vi "8.9.1.vi"() -> ()   [LabVIEW 2018]
panel:
  in  "정지":bool
  in  "데이터송신":bool
  out "수신 데이터":string
  in  "송신 데이터":string
  out "슬레이브 루프 반복":dbl
  out "마스터 루프 반복":dbl
  # "송신"
  # "송신안함"
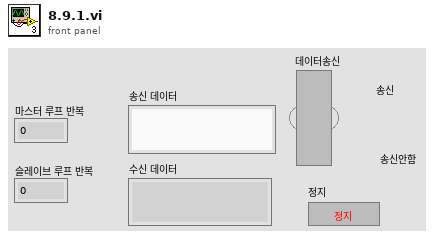
[diagram p1: front panel]
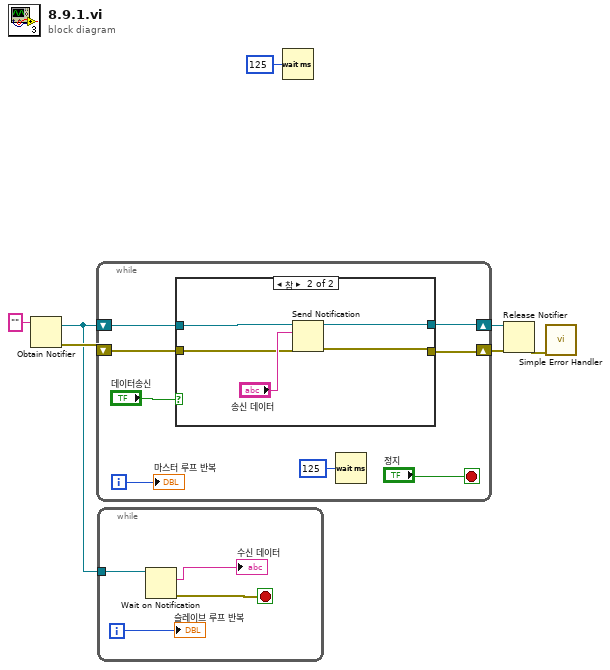
[diagram p0: block diagram]
diagram:
  n1 = Obtain Notifier(notification data type="" ("송신 데이터")) -> (notifier out=w1:refnum<notifier>, error out=w3:errorcluster)  [unwired: 3 in, 1 out]
  n2 = while {
    shift-right: [w11] -> w4
    shift-left: w1 -> [w12]
    shift-right: [w9] -> w2
    shift-left: w3 -> [w10]
    i -> [w15]
    stop <- "정지" stop-if-true
    n3 = case shown="참" "데이터송신" {
      tunnel: w12 -> [w17 w21]
      tunnel: [w17 w20] -> w11
      tunnel: w10 -> [w16 w19]
      tunnel: [w16 w18] -> w9
      frame False {
      }
      frame True {
        n4 = Send Notification(notification="송신 데이터", notifier=w21, error in (no error)=w19) -> (notifier out=w20:refnum<notifier>, error out=w18:errorcluster)
      }
    }
    n5 = Wait (ms)(milliseconds to wait=u32 125 ("대기 시간 (ms)")) -> ()  [unwired: 1 out]
    "마스터 루프 반복" <- w15
  }
  n6 = while {
    tunnel: w1 -> [w23]
    i -> [w26]
    stop <- w25 stop-if-true
    n7 = Wait on Notification(notifier=w23) -> (notification=→"수신 데이터":string, error out=w25:errorcluster)  [unwired: 3 in, 2 out]
    "슬레이브 루프 반복" <- w26
  }
  n8 = Wait (ms)(milliseconds to wait=u32 125 ("대기 시간 (ms)")) -> ()  [unwired: 1 out]
  n9 = Release Notifier(notifier=w4, error in (no error)=w2) -> (error out=w5:errorcluster)  [unwired: 1 in, 2 out]
  n10 = call <vilib>:"Simple Error Handler.vi"("error in (no error)"=w5) -> ()  [unwired: 4 in, 5 out]
